vi "data sample half(50ms).vi"(8 "Number of Remove data":i32, 9 "Offset":i32, 11 "Array":string[](array[string])) -> (3 "Array out":string[](array[string]))   [LabVIEW 2015]
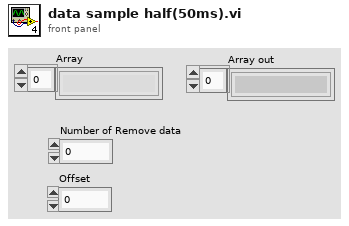
[diagram p1: front panel]
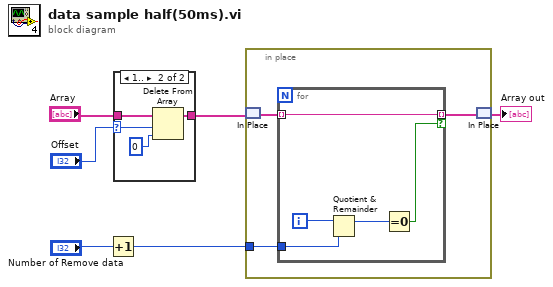
[diagram p0: block diagram]
diagram:
  n1 = Increment(x="Number of Remove data") -> (x+1=w4:i32)
  n2 = case shown="1.." "Offset" {
    selector: "Offset" -> [_ w9]
    tunnel: "Array" -> [w7 w11]
    tunnel: [w7 w10] -> w2
    frame 0, Default {
    }
    frame 1.. {
      n3 = Delete From Array(array=w11, length=w9, index=0 ("인덱스")) -> (array with subset deleted=w10:string[])  [unwired: 1 out]
    }
  }
  n4 = in-place {
    in-place-border: w4 -> [w12]
    n5 = in-place-match #1(w2) -> (w14:string[])
    n6 = for {
      tunnel: w14 -> [w15] mode=indexing
      tunnel: [w15] -> w13 mode=indexing if=w17
      tunnel: w12 -> [w16]
      i -> [w19]
      n7 = Quotient & Remainder(x=w19, y=w16) -> (x-y*floor(x/y)=w18:i32)  [unwired: 1 out]
      n8 = Equal To 0?(x=w18) -> (x = 0?=w17:bool)
    }
    n9 = in-place-match #1(w13) -> (→"Array out":string[])
  }
